vi "MAIN_merFISH_move_to_REF.vi"(0 "Data cluster":T1, 1 "queue piezo":refnum<queue>, 2 "queue ASI stage":refnum<queue>, 5 "ROI manager":i32(listbox), 9 "variant":variant, 11 "error in":errorcluster, 12 "XY positions Refnum":refnum<vi>, 13 "Global parameters IN":T2 {"# repetitions" min=0; "Dt (s)" min=0 step=1; "Filter list" items=["ET665lp", "zet405/488/561/640m", "None", "None", "None", "None"]}) -> (6 "XY positions OUT":dbl[][](array[numeric]), 8 "Next task":T3, 10 "XY graph":cluster{dbl[], dbl[]}[](array[cluster]), 14 "Global parameters out":T2 {"# repetitions" min=0; "Dt (s)" min=0 step=1; "Filter list" items=["ET665lp", "zet405/488/561/640m", "None", "None", "None", "None"]}, 15 "error out":errorcluster)   [LabVIEW 2015]
uses:
  CONTROLS/Q_ASI_stage_element.ctl
  CONTROLS/Q_MCL_piezo_element.ctl
  CONTROLS/Global parameters.ctl
  CONTROLS/Q_main_element.ctl
  GLOBAL/Global_MCL_piezo.vi
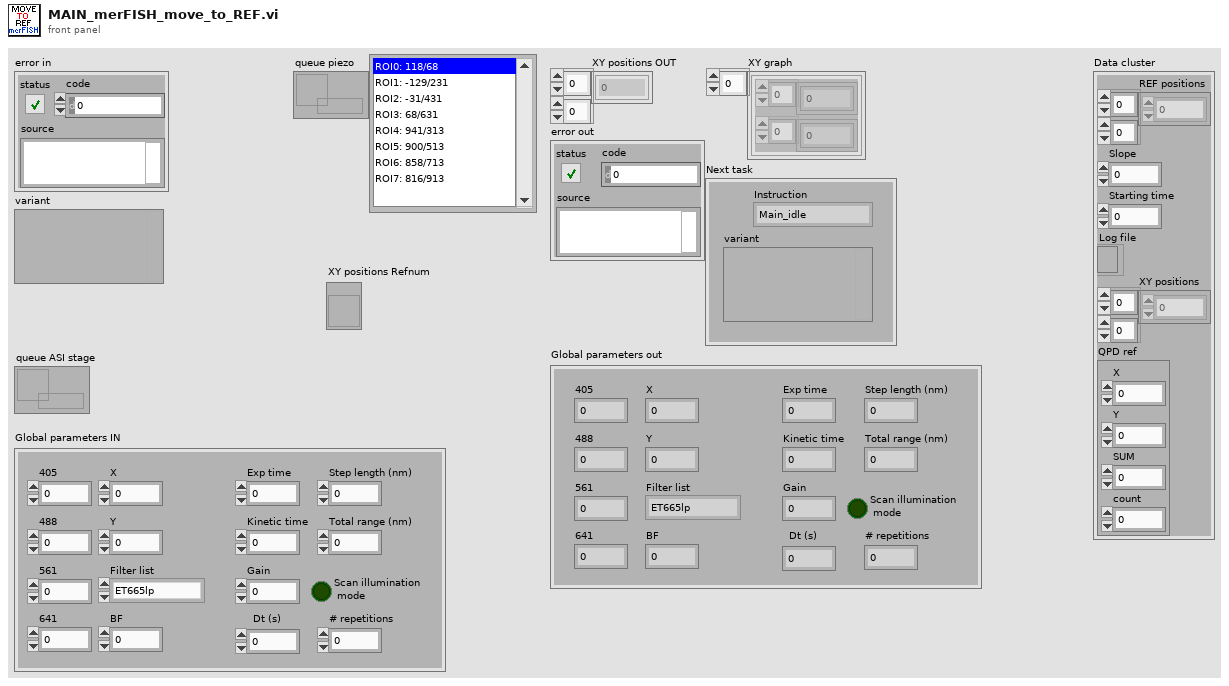
[diagram p1: front panel]
types:
  T1 = cluster{"REF positions":dbl[][], "Slope":dbl, "Starting time":dbl, "Log file":refnum<file>, "XY positions":dbl[][], "QPD ref":cluster{"X":sgl, "Y":sgl, "SUM":sgl, "count":u32}}
  T2 = typedef "Global parameters.ctl" = cluster{"405":dbl, "488":dbl, "561":dbl, "641":dbl, "BF":dbl, "X":dbl, "Y":dbl, "Filter list":u16, "Exp time":sgl, "Kinetic time":sgl, "Gain":i32, "Step length (nm)":u32, "Total range (nm)":u32, "Scan illumination\n mode":bool, "Dt (s)":i32, "# repetitions":i32}
  T3 = typedef "Q_main_element.ctl" = cluster{"variant":variant, "Instruction":enum16{"Main_idle", "Main_initialize", "Main_initialize_TDMS", "Main_initialize_Queue", "Main_error", "Main_DAQ_initialization_results", "Main_ASI_initialization_results", "Main_Piezo_initialization_results", "Main_Valve_initialization_results", "Main_Pump_initialization_results", "Main_CAMERA_initialization_results", "Main_FPGA_initialization_results", "Main_DAQ_error", "Main_ASI_error", "Main_Piezo_error", "Main_CAMERA_error", "Main_Valve_error", "Main_Pump_error", "Main_FPGA_error", "Main_start_acquiring", "Main_not_acquiring", "Main_acquiring", "Main_stop_acquiring", "Main_change_exposure", "Main_change_z_scan_parameters", "Main_define_ROI", "Main_define_mosaic", "Main_read_kinetic_time", "Main_cooler", "Main_read_temperature", "Main_save_XY", "Main_load_XY", "Main_discard_XY", "Main_move_to_XY", "Main_measure_QPD", "Main_autofocus_calibration", "Main_autofocus_initialization", "Main_autofocus_stop", "Main_save_PID", "Main_change_H_valve_position", "Main_two_way_valve", "Main_save_movie", "Main_init_single_scan", "Main_single_scan", "Main_stop_single_scan", "Main_merFISH_illumination_parameters", "Main_merFISH_buffer_probe_list", "Main_merFISH_injections_procedure", "Main_merFISH_save_setpoint", "Main_merFISH_DAPI_parameters", "Main_merFISH_Brightfield_parameters", "Main_merFISH_save_embryo_ROI", "Main_merFISH_init", "Main_merFISH_resume", "Main_merFISH_start_autofocus", "Main_merFISH_open_close_valve_merFISH", "Main_merFISH_open_close_valve_photobleaching", "Main_merFISH_hybridization", "Main_merFISH_move_to_ROI", "Main_merFISH_wait_stabilization", "Main_merFISH_move_to_REF", "Main_merFISH_scan", "Main_merFISH_photobleaching_injection", "Main_merFISH_photobleaching", "Main_merFISH_send_email", "Main_merFISH_close", "Main_STOP"}}
  T4 = cluster{"X":sgl, "Y":sgl, "SUM":sgl, "count":u32}
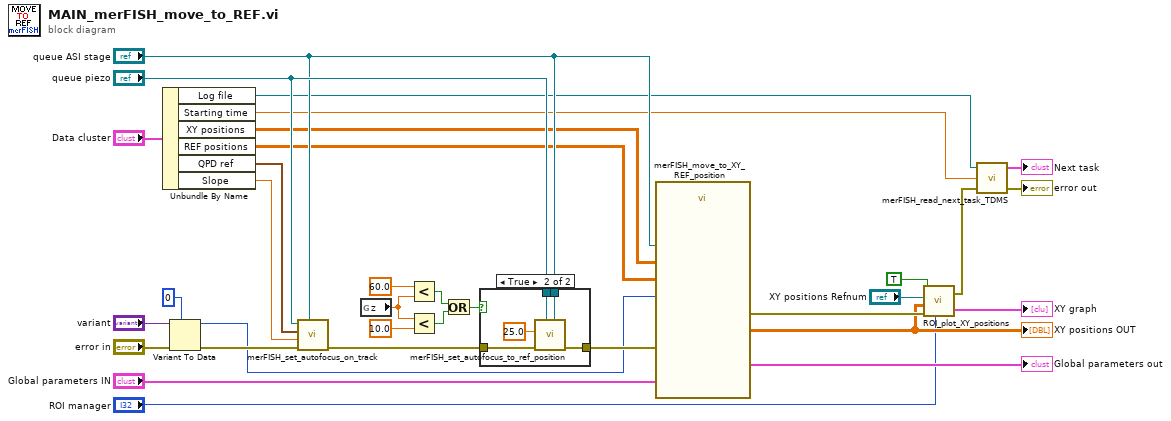
[diagram p0: block diagram]
diagram:
  n1 = Unbundle By Name("Data cluster") -> ("Log file"=w9:refnum<file>, "Starting time"=w8:dbl, "XY positions"=w6:dbl[][], "REF positions"=w7:dbl[][], "QPD ref"=w4:T4, "Slope"=w18:dbl)
  n2 = Variant To Data(error in="error in", type=0 ("ROI #"), Variant="variant") -> (data=w1:i32, error out=w24:errorcluster)
  n3 = call "merFISH_set_autofocus_on_track.vi"("queue ASI stage"="queue ASI stage", "error in"=w24, "Slope"=w18, "QPD ref"=w4, "queue piezo"="queue piezo") -> ("error out"=w26:errorcluster)  [unwired: 4 in]
  n4 = global read "Global_MCL_piezo.vi" "z"() -> (w29:dbl)
  n5 = Less?(x=60.0, y=w29) -> (x < y?=w31:bool)
  n6 = Less?(x=w29, y=10.0) -> (x < y?=w32:bool)
  n7 = Or(x=w31, y=w32) -> (x .or. y?=w33:bool)
  n8 = case shown="True" w33 {
    tunnel: w26 -> [w34 w38]
    tunnel: [w34 w37] -> w27
    tunnel: "queue piezo" -> [_ w36]
    tunnel: "queue ASI stage" -> [_ w35]
    frame False {
    }
    frame True {
      n9 = call "merFISH_set_autofocus_to_ref_position.vi"("queue ASI stage"=w35, "queue piezo"=w36, "error in"=w38, "Ref"=25.0) -> ("error out"=w37:errorcluster)  [unwired: 7 in]
    }
  }
  n10 = call "merFISH_move_to_XY_REF_position.vi"("REF #"=w1, "Global parameters"="Global parameters IN", "XY positions"=w6, "queue ASI stage"="queue ASI stage", "error in"=w27, "REF positions"=w7) -> ("Global parameters out"=→"Global parameters out":T2, "error out"=w25:errorcluster, "XY positions"=w23:dbl[][])  [unwired: 3 in]
  "XY positions OUT" <- w23
  n11 = call "ROI_plot_XY_positions.vi"("Display?"=TRUE, "XYGraph Refnum"="XY positions Refnum", "XY positions"=w23, "error in"=w25, "ROI manager"="ROI manager") -> ("error out"=w3:errorcluster, "XY graph"=→"XY graph":cluster{dbl[], dbl[]}[])
  n12 = call "merFISH_read_next_task_TDMS.vi"("error in"=w3, "Starting time"=w8, "Log file"=w9) -> ("error out"=→"error out":errorcluster, "task"=→"Next task":T3)  [unwired: 1 in]
